vi "Bezier Curve.vi"(9 "position":sgl[](array[numeric]), 10 "percision":sgl, 11 "ctrl points":cluster{sgl, sgl}[](array[cluster])) -> (2 "position out":sgl[](array[numeric]), 3 "curve":T1)   [LabVIEW 2025]
uses:
  Types/Bezier Curve.ctl
  <vilib>/Analysis/2dsp.llb/2D Inverse Complex FFT.vi
  <vilib>/Analysis/NI_AALPro.lvlib
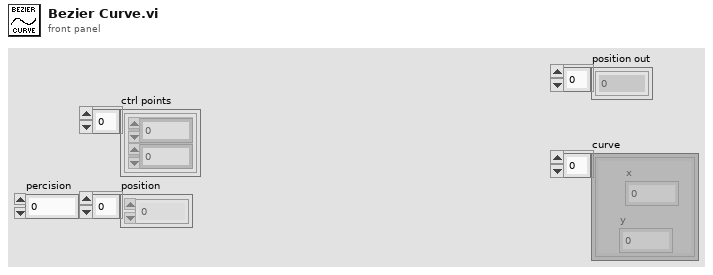
[diagram p1: front panel]
types:
  T1 = typedef "Bezier Curve.ctl" = cluster{"x":sgl, "y":sgl}[]
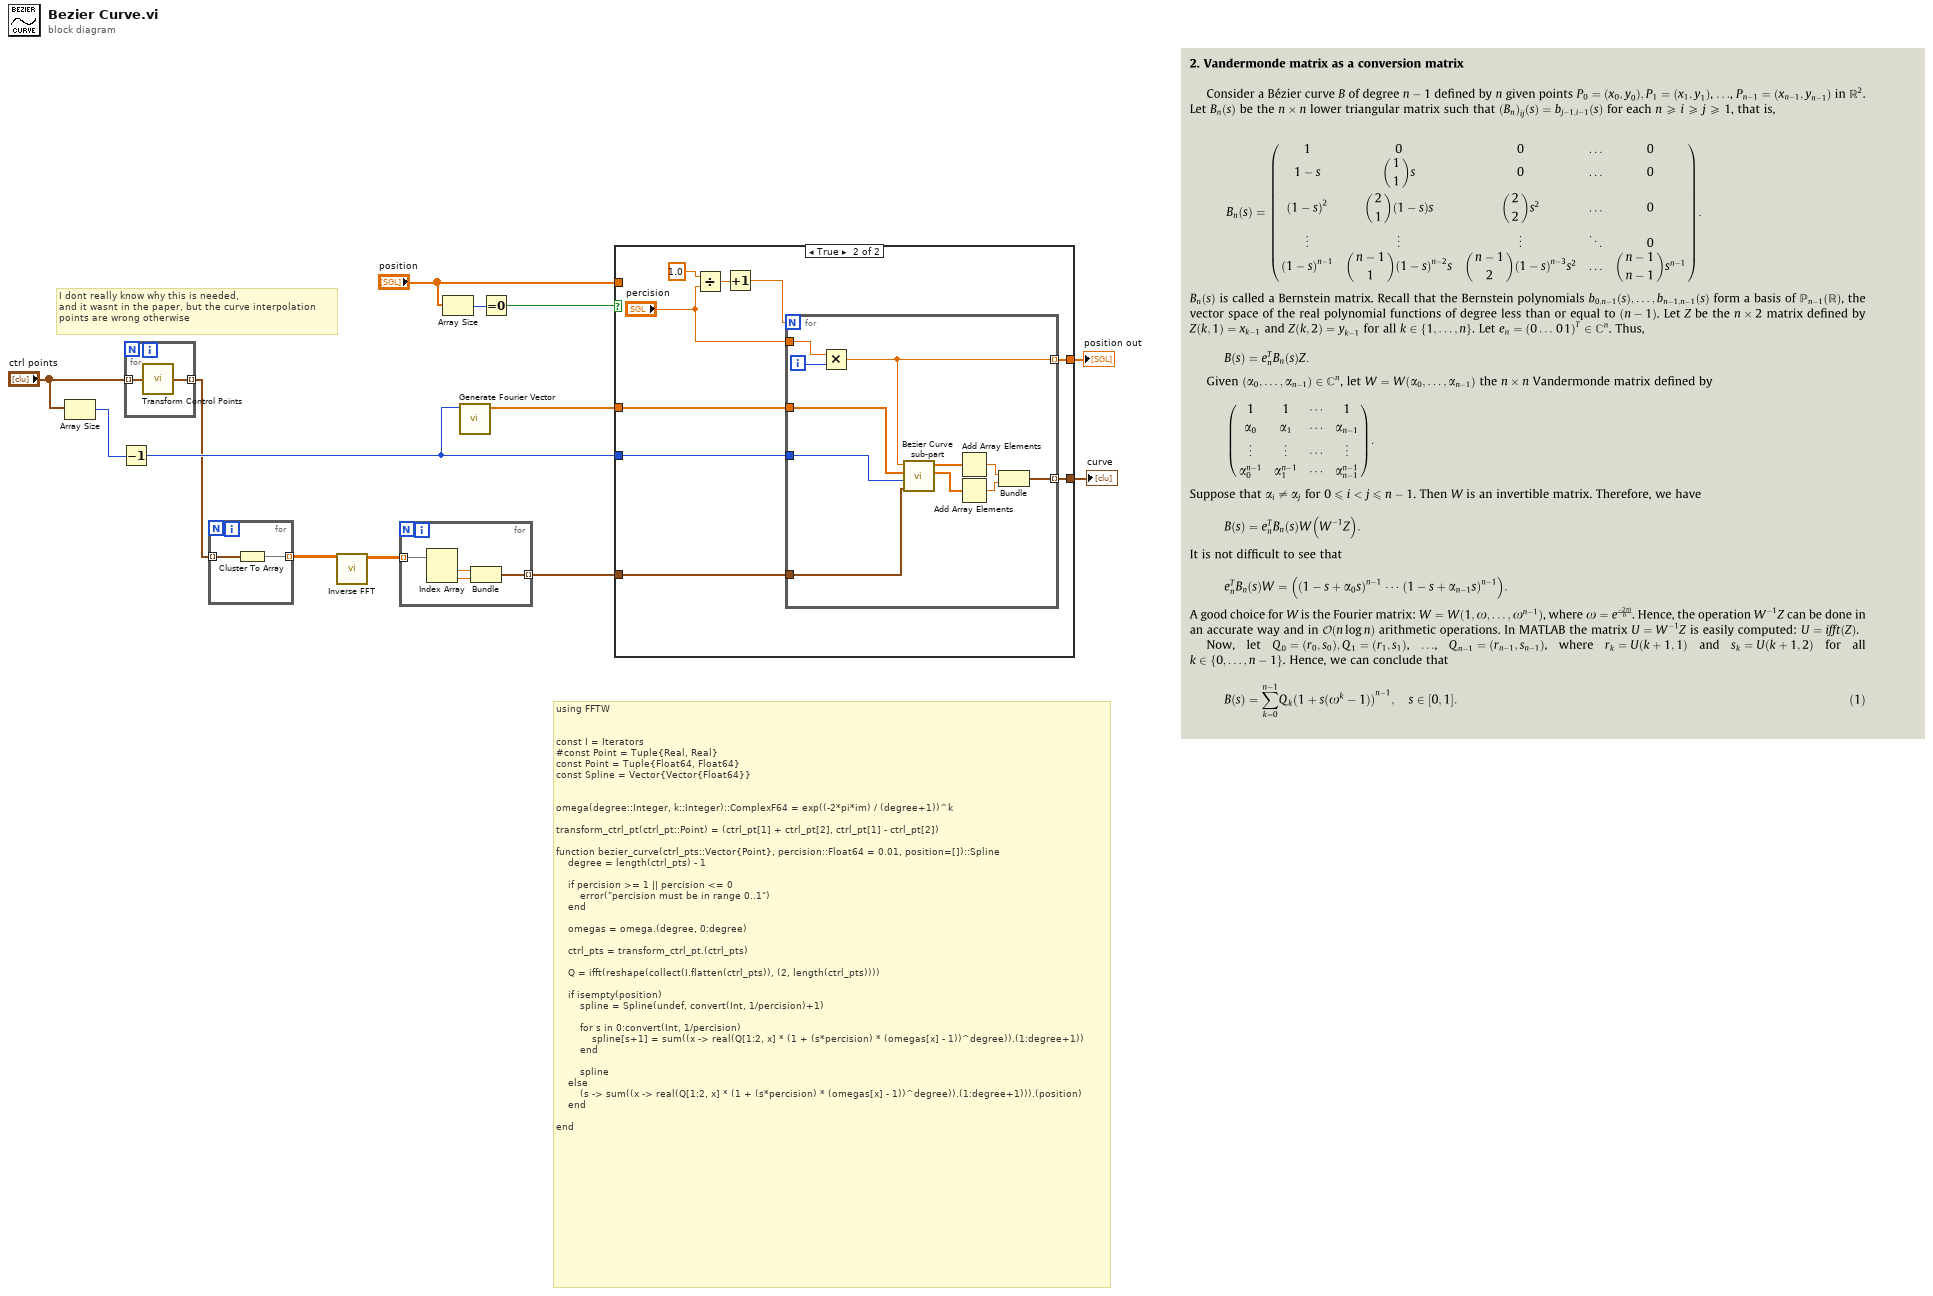
[diagram p0: block diagram]
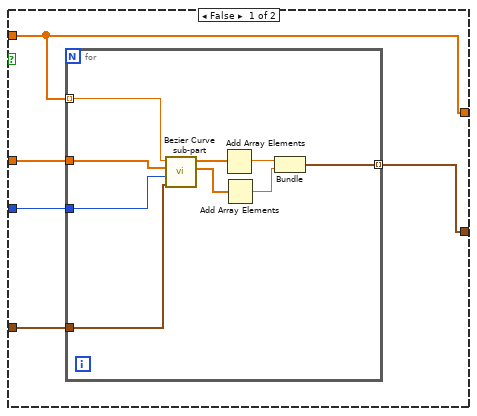
[diagram p2: hidden frame]
diagram:
  # "I dont really know why this is needed,\nand it wasnt in the paper, but the curve interpolation\npoints are wrong otherwise"
  # "using FFTW\n\n\nconst I = Iterators\n#const Point = Tuple{Real, Real}\nconst Point = Tuple{Float64, Float64}\nconst Spline = Vector{Vector{Float64}}\n\n\nomega(degree::Integer, k::Integer)::ComplexF64 = exp((-2*pi*im) / (degree+1))^k\n\ntransform_ctrl_pt(ctrl_pt::Point) = (ctrl_pt[1] + ctrl_pt[2], ctrl_pt[1] - ctrl_pt[2])\n\nfunction bezier_curve(ctrl_pts::Vector{Point}, percision::Float64 = 0.01, position=[])::Spline\n    degree = length(ctrl_pts) - 1\n\n    if percision >= 1 || percision <= 0\n        error(\"percision must be in range 0..1\")\n    end\n\n    omegas = omega.(degree, 0:degree)\n\n    ctrl_pts = transform_ctrl_pt.(ctrl_pts)\n\n    Q = ifft(reshape(collect(I.flatten(ctrl_pts)), (2, length(ctrl_pts))))\n\n    if isempty(position)\n        spline = Spline(undef, convert(Int, 1/percision)+1)\n\n        for s in 0:convert(Int, 1/percision)\n            spline[s+1] = sum((x -> real(Q[1:2, x] * (1 + (s*percision) * (omegas[x] - 1))^degree)).(1:degree+1))\n        end\n\n        spline\n    else\n        (s -> sum((x -> real(Q[1:2, x] * (1 + (s*percision) * (omegas[x] - 1))^degree)).(1:degree+1))).(position)\n    end\n\nend"
  n1 = Array Size(array="ctrl points") -> (size(s)=w7:i32)
  n2 = Decrement(x=w7) -> (x-1=w6:i32)
  n3 = for {
    tunnel: "ctrl points" -> [w15] mode=indexing
    tunnel: [w14] -> w5 mode=indexing
    n4 = call "Transform Control Points.vi"("ctrl pt"=w15) -> ("ctrl pt out"=w14:cluster{dbl, dbl})
  }
  n5 = for {
    tunnel: w5 -> [w17] mode=indexing
    tunnel: [w16] -> w13 mode=indexing
    n6 = Cluster To Array(cluster=w17) -> (array=w16:dbl[])
  }
  n7 = call-poly <vilib>:"Inverse FFT.vi"("FFT {x}"=w13) -> ("X"=w12:cdb[][])  [unwired: 9 in, 1 out]
  n8 = for {
    tunnel: w12 -> [w21] mode=indexing
    tunnel: [w18] -> w11 mode=indexing
    n9 = Index Array(array=w21) -> (element #1=w20:cdb, element #2=w19:cdb)  [unwired: 2 in]
    n10 = Bundle(w20, w19) -> (w18:cluster{cdb, cdb})  [unwired: 1 in]
  }
  n11 = Array Size(array="position") -> (size(s)=w4:i32)
  n12 = call "Generate Fourier Vector.vi"("degree"=w6) -> ("Fourier Matrix"=w9:cdb[])  [unwired: 10 in]
  n13 = Equal To 0?(x=w4) -> (x = 0?=w3:bool)
  n14 = case shown="True" w3 {
    tunnel: w11 -> [w24 w43]
    tunnel: [w23 w42] -> w10
    tunnel: w9 -> [w26 w41]
    tunnel: w6 -> [w25 w38]
    tunnel: "position" -> [w22 _]
    tunnel: [w22 w36] -> w1
    frame False {
      n15 = for {
        tunnel: w22 -> [w35] mode=indexing
        tunnel: w26 -> [w34]
        tunnel: w25 -> [w33]
        tunnel: w24 -> [w32]
        tunnel: [w27] -> w23 mode=indexing
        n16 = call "Bezier Curve sub-part.vi"("Q"=w32, "degree"=w33, "Fourier Matrix"=w34, "position"=w35) -> ("y arr"=w30:dbl[], "x arr"=w31:dbl[])  [unwired: 6 in]
        n17 = Add Array Elements(numeric array=w31) -> (sum=w29:dbl)
        n18 = Add Array Elements(numeric array=w30) -> (sum=w28:dbl)
        n19 = Bundle(w29, w28) -> (w27:cluster{dbl, dbl})  [unwired: 1 in]
      }
    }
    frame True {
      n20 = Divide(x=1.0, y="percision") -> (x/y=w40:dbl)
      n21 = Increment(x=w40) -> (x+1=w39:dbl)
      n22 = for {
        N: w39 -> [_]
        tunnel: "percision" -> [w49]
        tunnel: w38 -> [w47]
        tunnel: w43 -> [w46]
        tunnel: [w50] -> w42 mode=indexing
        tunnel: w41 -> [w48]
        tunnel: [w45] -> w36 mode=indexing
        i -> [w55]
        n23 = Multiply(x=w49, y=w55) -> (x*y=w45:sgl)
        n24 = call "Bezier Curve sub-part.vi"("Q"=w46, "degree"=w47, "Fourier Matrix"=w48, "position"=w45) -> ("y arr"=w53:dbl[], "x arr"=w54:dbl[])  [unwired: 6 in]
        n25 = Add Array Elements(numeric array=w54) -> (sum=w51:dbl)
        n26 = Add Array Elements(numeric array=w53) -> (sum=w52:dbl)
        n27 = Bundle(w51, w52) -> (w50:cluster{dbl, dbl})  [unwired: 1 in]
      }
    }
  }
  "curve" <- w10
  "position out" <- w1
